vi "Is Binning Available.vi"(8 "error in (no error)":errorcluster, 11 "Camera in":refnum<class "Camera.lvclass">) -> (0 "error out":errorcluster, 2 "Avaliable":bool, 3 "Camera":refnum<class "Camera.lvclass">)   [LabVIEW 2020, in "Camera.lvclass"]
uses:
  Camera.lvclass
  Camera.lvclass/Camera.ctl
  bin/gindustrialcam_32-1.dll
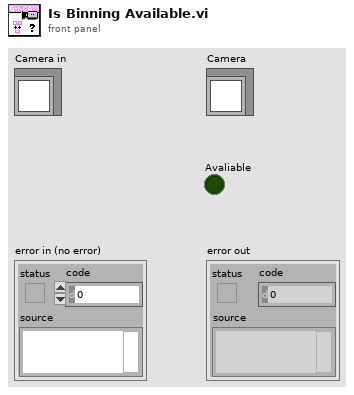
[diagram p1: front panel]
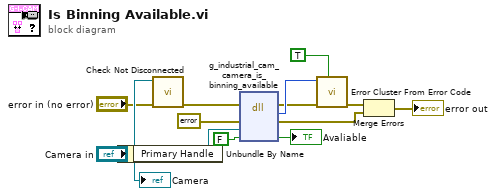
[diagram p0: block diagram]
diagram:
  n1 = Unbundle By Name("Camera in") -> ("Primary Handle"=w8:refnum<data-value>)
  n2 = call "Check Not Disconnected.vi"("error in (no error)"="error in (no error)", "Camera in"="Camera in") -> ("error out"=w9:errorcluster)  [unwired: 9 in]
  n3 = dll-call lib="C:/serenial/lib/g-industrial-camera/LabVIEW/g_industrial_cam/bin/gindustrialcam_*-1.*" fn="g_industrial_cam_camera_is_binning_available"(error in=w9, "err"=errorcluster {"status"=FALSE, "code"=0, "source"=""} ("error constant"), "edvr"=w8, "available"=FALSE ("Set?")) -> (error out=w2:errorcluster, "Mg_Error"=w3:i32, "err"=w5:errorcluster, "available"=→"Avaliable":bool)  [unwired: 3 in, 1 out]
  n4 = call <vilib>:"Error Cluster From Error Code.vi"("show call chain? (False)"=TRUE, "error in (no error)"=w2, "error code (0)"=w3) -> ("error out"=w4:errorcluster)  [unwired: 6 in]
  n5 = Merge Errors(w4, w5) -> (→"error out":errorcluster)
  "Camera" <- "Camera in"
